vi "Read Key (Raw).vi"(7 "Section Name":string, 8 "error in (no error)":errorcluster, 10 "Key Name":string, 11 "Config in":T1) -> (0 "error out":errorcluster, 1 "Content":string, 2 "Key Found?":bool, 3 "Config out":T1)   [LabVIEW 2022 SP3, in "LabVIEW-Config.lvlib"]
uses:
  LabVIEW-Config.lvlib
  Config.ctl
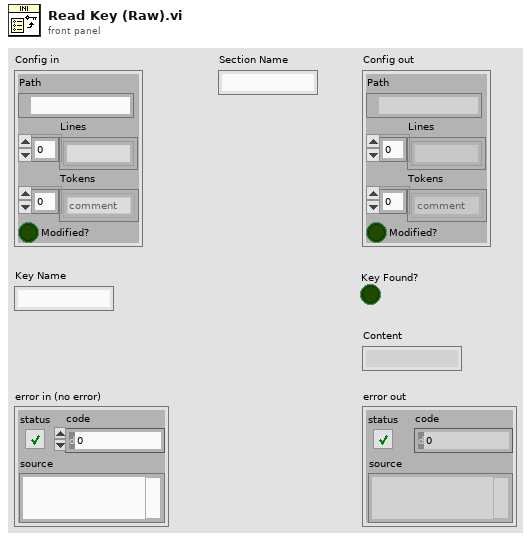
[diagram p1: front panel]
types:
  T1 = typedef "LabVIEW-Config.lvlib/Config.ctl" = cluster{"Path":path, "Lines":string[], "Tokens":enum8{"comment", "section", "key"}[], "Modified?":bool}
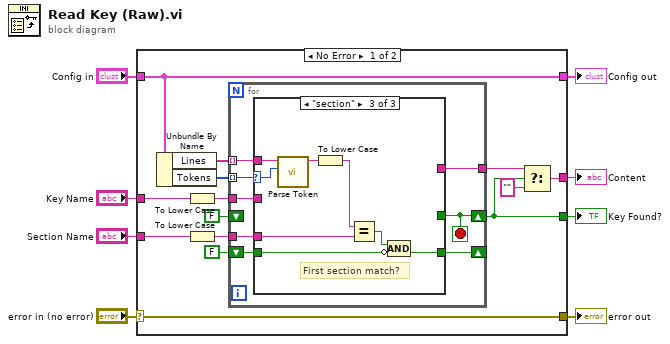
[diagram p0: block diagram]
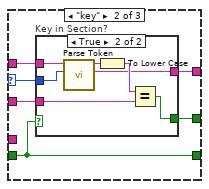
[diagram p3: hidden frame]
diagram:
  n1 = case shown="No Error" "error in (no error)" {
    selector: "error in (no error)" -> [w21 w54]
    tunnel: "Config in" -> [w16 w53]
    tunnel: [w21 w54] -> w7
    tunnel: [w16 w53] -> w5
    tunnel: "Section Name" -> [w20 _]
    tunnel: [w13 _] -> w3
    tunnel: "Key Name" -> [w15 _]
    tunnel: [w9 _] -> w1
    frame No Error {
      n2 = Unbundle By Name(w16) -> ("Lines"=w22:string[], "Tokens"=w10:enum8{"comment", "section", "key"}[])
      n3 = To Lower Case(string=w15) -> (all lower case string=w14:string)
      n4 = To Lower Case(string=w20) -> (all lower case string=w19:string)
      n5 = for {
        tunnel: w10 -> [w30] mode=indexing
        tunnel: w22 -> [w29] mode=indexing
        tunnel: w19 -> [w28]
        shift-right: [w26] -> _
        shift-left: FALSE -> [w27]
        shift-right: [w24] -> w13
        shift-left: FALSE -> [_]
        tunnel: w14 -> [w25]
        tunnel: [w23] -> w12
        stop <- w24 stop-if-true
        n6 = case shown="\"section\"" w30 {
          selector: w30 -> [_ w32 w46]
          tunnel: w29 -> [_ w37 w47]
          tunnel: w28 -> [_ _ w52]
          tunnel: [w31 w36 w48] -> w26
          tunnel: w27 -> [w31 w36 w50]
          tunnel: w25 -> [_ w35 _]
          tunnel: [_ w34 _] -> w24
          tunnel: [_ w33 _] -> w23
          frame "comment" {
          }
          frame "key" {
            n7 = case "Key in Section?" shown="True" w36 {
              tunnel: w37 -> [_ w41]
              tunnel: w35 -> [_ w44]
              tunnel: [_ w42] -> w34
              tunnel: [_ w38] -> w33
              tunnel: w32 -> [_ w40]
              frame False {
              }
              frame True {
                n8 = call "Parse Token.vi"("Token"=w40, "Line"=w41) -> ("Value"=w38:string, "Name"=w39:string)  [unwired: 8 in]
                n9 = To Lower Case(string=w39) -> (all lower case string=w43:string)
                n10 = Equal?(x=w43, y=w44) -> (x = y?=w42:bool)
              }
            }
          }
          frame "section" {
            # "First section match?"
            n11 = call "Parse Token.vi"("Token"=w46, "Line"=w47) -> ("Name"=w45:string)  [unwired: 8 in, 1 out]
            n12 = To Lower Case(string=w45) -> (all lower case string=w51:string)
            n13 = Equal?(x=w51, y=w52) -> (x = y?=w49:bool)
            n14 = Compound Arithmetic op=AND(w49, invert w50) -> (w48:bool)
          }
        }
      }
      n15 = Select(t=w12, s=w13, f="") -> (s? t:f=w9:string)
    }
    frame Error {
    }
  }
  "error out" <- w7
  "Config out" <- w5
  "Key Found?" <- w3
  "Content" <- w1
